vi "test Import-Script-Deploy.vi"(8 "error in":errorcluster, 11 "Import-Script-Deploy.lvclass":refnum<class "Import-Script-Deploy.lvclass">) -> (0 "error out":errorcluster, 3 "Import-Script-Deploy.lvclass":refnum<class "Import-Script-Deploy.lvclass">)   [LabVIEW 2020, in "Import-Script-Deploy.lvclass"]
uses:
  Import-Script-Deploy.lvclass
  <vilib>/addons/_JKI Toolkits/VI Tester/TestCase.llb/TestCase.lvclass
  4b06c685-66bb-4135-9ad1-d89a50a95502.vi
  Import/ARINC 429 Import.lvlib
  Scripting/Ballard ARINC 429 Scripting.lvlib
  Shared/Initialization Method.ctl
  Shared/Device Parameters.ctl
  niveristand-custom-device-testing-tools/VeriStandTestUtilities/VeriStandTestUtilities.lvlib
  C:/Program Files (x86)/National Instruments/LabVIEW 2020/vi.lib/addons/_JKI Toolkits/VI Tester/TestCase.llb/TestCase.lvclass
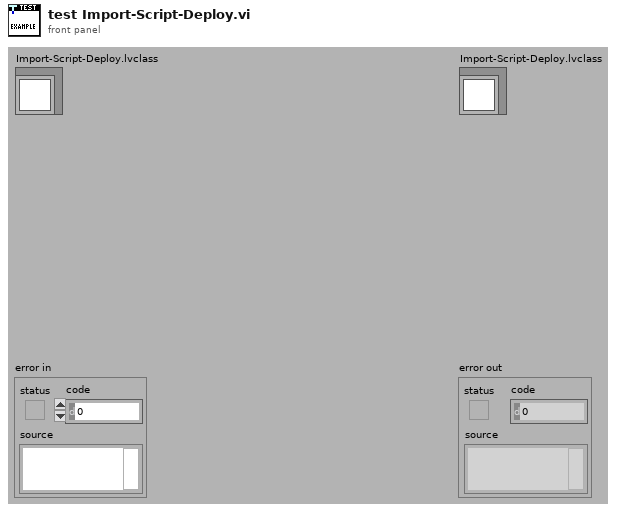
[diagram p1: front panel]
types:
  T1 = typedef "Device Parameters.ctl" = cluster{"initialization method":T2, "card number":i32, "PXI slot number":i32, "core number":i32}
  T2 = typedef "Initialization Method.ctl" = enum16{"PXI Slot Number", "Card Number"}
  T3 = typedef "VS Channels Definition for All Labels on Hardware Channel.ctl" = cluster{"hardware channel":i32, "labels":T4[]}
  T4 = typedef "VS Channels Definition for Label.ctl" = cluster{"label (Dec)":u32, "parameters":T5[], "SDI value":u8, "SDI enabled":bool, "transfer type":T9}
  T5 = typedef "VS Channel Definition for Parameter.ctl" = cluster{"name":string, "direction":T6, "default value":dbl, "unit":string, "Parameter":T7}
  T6 = typedef "Direction.ctl" = enum16{"Rx", "Tx"}
  T7 = typedef "Parameter Definition.ctl" = cluster{"start index":i32, "size":i32, "encoding":T8, "signed":bool, "scale multiplier":dbl, "scale offset":dbl}
  T8 = typedef "Encoding and Decoding.lvlib/Encoding.ctl" = enum16{"BNR", "BCD", "Discrete"}
  T9 = typedef "Transfer Type.ctl" = enum16{"Scheduled", "Acyclic", "Block", "Strobe"}
  T10 = typedef "Custom Device API.lvlib/Custom Device Item Ref.ctl" = u64
  T11 = typedef "NI_VS Workspace ExecutionAPI.lvlib/WorkspaceAPI.ctl" = refnum<k24>
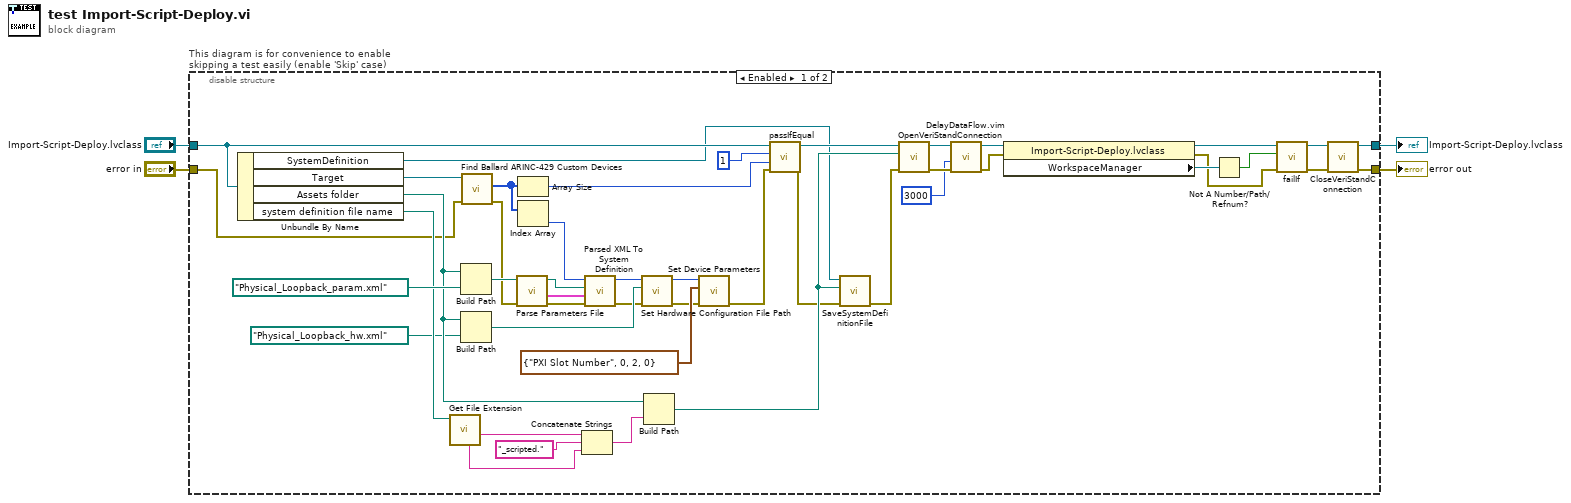
[diagram p0: block diagram]
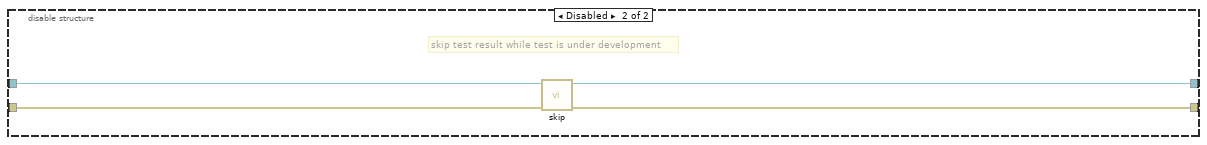
[diagram p2: hidden frame]
diagram:
  n1 = disable-structure "This diagram is for convenience to enable skipping a test easily (enable 'Skip' case)" shown="Enabled" {
    disable-tunnel: "Import-Script-Deploy.lvclass" -> [w35 w52]
    disable-tunnel: [w47 w51] -> w3
    disable-tunnel: "error in" -> [w6 w50]
    disable-tunnel: [w37 w49] -> w1
    frame Enabled {
      n2 = Unbundle By Name(w35) -> ("SystemDefinition"=w7:refnum<k24>, "Target"=w36:refnum<k24>, "Assets folder"=w16:path, "system definition file name"=w24:path)
      n3 = call <vilib>:"Get File Extension.vi"("file"=w24) -> ("filename without extension"=w23:string, "unmodified file extension"=w21:string)  [unwired: 6 in, 3 out]
      n4 = Build Path(base path=w16, name or relative path=path "Physical_Loopback_param.xml" ("Absolute or Relative Path")) -> (appended path=w40:path)
      n5 = Build Path(base path=w16, name or relative path=path "Physical_Loopback_hw.xml" ("Absolute or Relative Path")) -> (appended path=w14:path)
      n6 = call "Find Ballard ARINC-429 Custom Devices.vi"("error in"=w6, "target in"=w36) -> ("error out"=w31:errorcluster, "Ballard ARINC 429 custom devices"=w5:u64[])  [unwired: 7 in, 1 out]
      n7 = call "Parse Parameters File.vi"("error in"=w31, "path to XML document"=w40) -> ("error out"=w39:errorcluster, "ports"=w38:T3[], "path to XML document out"=w13:path)  [unwired: 7 in]
      n8 = Array Size(array=w5) -> (size(s)=w34:i32)
      n9 = Index Array(array=w5) -> (element=w32:u64)  [unwired: 1 in]
      n10 = Concatenate Strings(w23, "_scripted." ("string"), w21) -> (w20:string)
      n11 = call "Parsed XML To System Definition.vi"("error in"=w39, "ports"=w38, "parameter configuration file path"=w13, "custom device ref"=w32) -> ("error out"=w11:errorcluster, "custom device ref out"=w12:T10)  [unwired: 6 in]
      n12 = call "Set Hardware Configuration File Path.vi"("error in"=w11, "path"=w14, "custom device ref"=w12) -> ("error out"=w9:errorcluster, "custom device ref out"=w10:T10)  [unwired: 7 in]
      n13 = Build Path(base path=w16, name or relative path=w20) -> (appended path=w19:path)
      n14 = call "Set Device Parameters.vi"("error in"=w9, "device parameters"=T1 {"initialization method"=enum."PXI Slot Number", "card number"=0, "PXI slot number"=2, "core number"=0}, "Ballard ARINC 429 custom device in"=w10) -> ("error out"=w8:errorcluster)  [unwired: 7 in, 1 out]
      n15 = call-dynamic "passIfEqual.vi"("error in (no error)"=w8, "y"=w34, "x"=1 ("size(s)"), "TestCase in"=w35) -> ("error out"=w17:errorcluster, "TestCase out"=w30:refnum<class "Import-Script-Deploy.lvclass">)  [unwired: 6 in]
      n16 = call "SaveSystemDefinitionFile.vi"("error in (no error)"=w17, "System Definition File in"=w19, "System Definition Reference in"=w7) -> ("error out"=w18:errorcluster)  [unwired: 7 in, 1 out]
      n17 = call-dynamic "OpenVeriStandConnection.vi"("error in (no error)"=w18, "System Definition File"=w19, "VeriStand Test Case in"=w30) -> ("error out"=w29:errorcluster, "VeriStand Test Case out"=w28:refnum<class "Import-Script-Deploy.lvclass">)  [unwired: 6 in, 1 out]
      n18 = call "DelayDataFlow.vim"("value in"=w29, "milliseconds to wait"=u32 3000) -> ("value out"=w48:errorcluster)  [unwired: 2 in, 1 out]
      n19 = property class="Import-Script-Deploy.lvclass"(reference=w28, error in=w48) -> (reference out=w46:refnum<class "Import-Script-Deploy.lvclass">, error out=w41:errorcluster, "WorkspaceManager"=w43:T11)
      n20 = Not A Number/Path/Refnum?(number/path/refnum=w43) -> (NaN/Path/Refnum?=w42:bool)
      n21 = call-dynamic "failIf.vi"("error in (no error)"=w41, "fail"=w42, "TestCase in"=w46) -> ("error out"=w44:errorcluster, "TestCase out"=w45:refnum<class "Import-Script-Deploy.lvclass">)  [unwired: 7 in]
      n22 = call-dynamic "CloseVeriStandConnection.vi"("error in (no error)"=w44, "VeriStand Test Case in"=w45) -> ("error out"=w47:errorcluster, "VeriStand Test Case out"=w37:refnum<class "Import-Script-Deploy.lvclass">)  [unwired: 8 in]
    }
    frame Disabled {
      # "skip test result while test is under development"
      n23 = call <vilib>:"skip.vi"("error in (no error)"=w50, "TestCase in"=w52) -> ("error out"=w51:errorcluster, "TestCase out"=w49:refnum<class "Import-Script-Deploy.lvclass">)  [unwired: 8 in]
    }
  }
  "error out" <- w3
  "Import-Script-Deploy.lvclass" <- w1
